vi "ShortestDistanceBetweenRegimesTest.vi"() -> (3 "Were there any errors at all?":bool)   [LabVIEW 2013]
uses:
  Data/TypeDefs/Sailing Regimes.ctl
panel:
  in  "Current regime inputs":T1[](array[typedef])=[enum."Upwind - Port Tack", enum."Upwind - Starboard Tack", enum."Reach - Port Tack", enum."Run - Starboard Tack", enum."Run - Port Tack", enum."Reach - Port Tack"]
  in  "Desired regime inputs":T1[](array[typedef])=[enum."Upwind - Port Tack", enum."Upwind - Starboard Tack", enum."Reach - Port Tack", enum."Run - Starboard Tack", enum."Run - Port Tack", enum."Reach - Port Tack"]
  in  "Expected regime outputs":T1[](array[typedef])=[enum."Upwind - Port Tack", enum."Upwind - Starboard Tack", enum."Reach - Port Tack", enum."Run - Starboard Tack", enum."Run - Port Tack", enum."Reach - Port Tack"]
  out "Actual regime outputs":T1[](array[typedef])=[enum."Upwind - Port Tack", enum."Upwind - Starboard Tack", enum."Reach - Port Tack", enum."Run - Starboard Tack", enum."Run - Port Tack", enum."Reach - Port Tack"]
  out "Are chosen regimes right?":bool[](array[boolean])=[TRUE, TRUE, TRUE, TRUE, TRUE, TRUE]
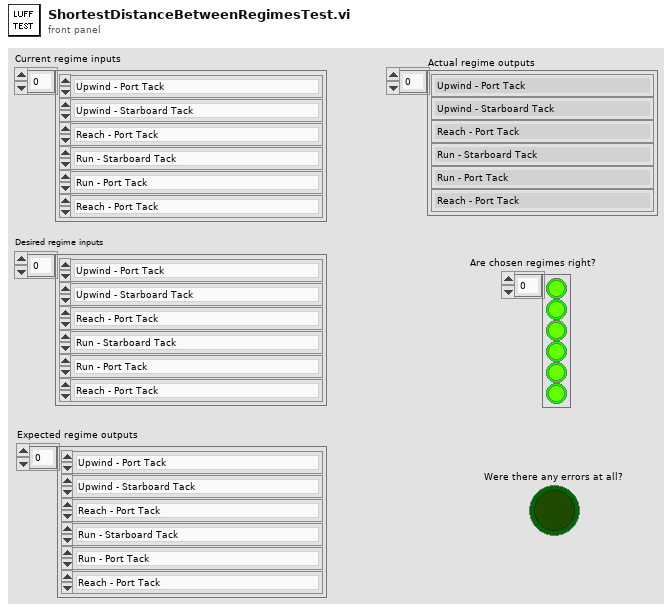
[diagram p1: front panel]
types:
  T1 = typedef "Sailing Regimes.ctl" = enum16{"Tack - Bow across wind", "Upwind - Starboard Tack", "Turn between Upwind/Reach - Starboard Tack", "Reach - Starboard Tack", "Turn between Reach/Run - Starboard Tack", "Run - Starboard Tack", "Jibe - Stern across wind", "Run - Port Tack", "Turn between Reach/Run - Port Tack", "Reach - Port Tack", "Turn between Upwind/Reach - Port Tack", "Upwind - Port Tack"}
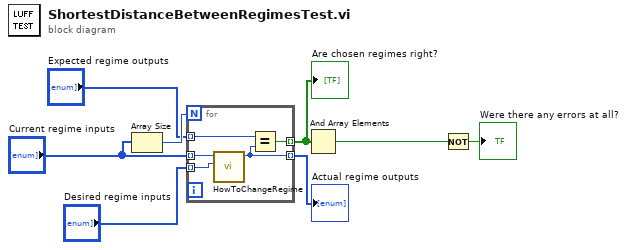
[diagram p0: block diagram]
diagram:
  n1 = Array Size(array="Current regime inputs") -> (size(s)=w8:i32)
  n2 = for {
    N: w8 -> [_]
    tunnel: "Expected regime outputs" -> [w13] mode=indexing
    tunnel: [w12] -> w7 mode=indexing
    tunnel: "Current regime inputs" -> [w10] mode=indexing
    tunnel: [w11] -> w3 mode=indexing
    tunnel: "Desired regime inputs" -> [w9] mode=indexing
    n3 = call "HowToChangeRegime.vi"("Desired Sailing Regime"=w9, "Current Sailing Regime"=w10) -> ("Output sailing regime"=w11:T1)  [unwired: 9 in]
    n4 = Equal?(x=w13, y=w11) -> (x = y?=w12:bool)
  }
  "Are chosen regimes right?" <- w7
  "Actual regime outputs" <- w3
  n5 = And Array Elements(Boolean array=w7) -> (logical AND=w5:bool)
  n6 = Not(x=w5) -> (.not. x?=→"Were there any errors at all?":bool)
